vi "m4.vi"(2 "input":string, 3 "file":string="Sequencer.m4") -> (0 "output":string)   [LabVIEW 2014]
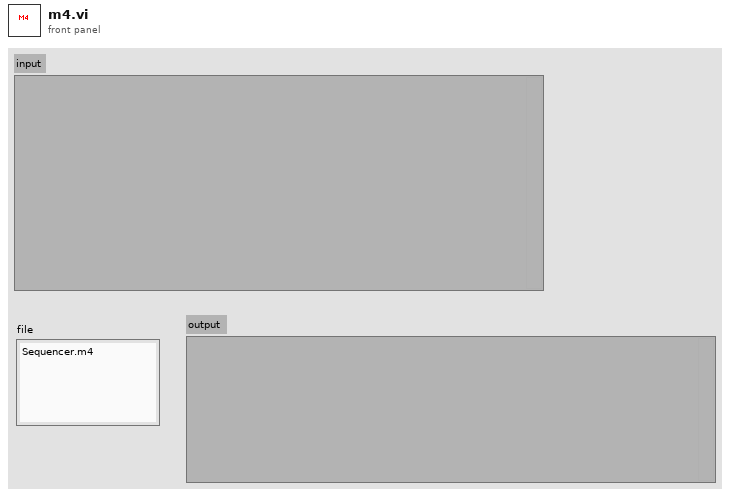
[diagram p1: front panel]
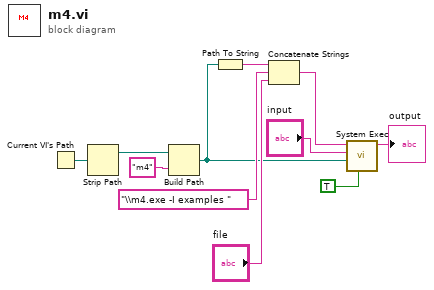
[diagram p0: block diagram]
diagram:
  n1 = Current VI's Path() -> (path=w4:path)
  n2 = Strip Path(path=w4) -> (stripped path=w3:path)  [unwired: 1 out]
  n3 = Build Path(base path=w3, name or relative path="m4") -> (appended path=w1:path)
  n4 = Path To String(path=w1) -> (string=w5:string)
  n5 = Concatenate Strings(w5, "\\m4.exe -I examples " ("command line"), "file") -> (w9:string)
  n6 = call <vilib>:"System Exec.vi"("run minimized? (F)"=TRUE, "working directory"=w1, "standard input"="input", "command line"=w9) -> ("standard output"=→"output":string)  [unwired: 4 in, 3 out]
